vi "TCP IP Connection Tester.vi"() -> ()   [LabVIEW 2024]
panel:
  out "Array":T1(array[cluster])
  in  "port":u16[](array[numeric])
  in  "address":string[](array[string])
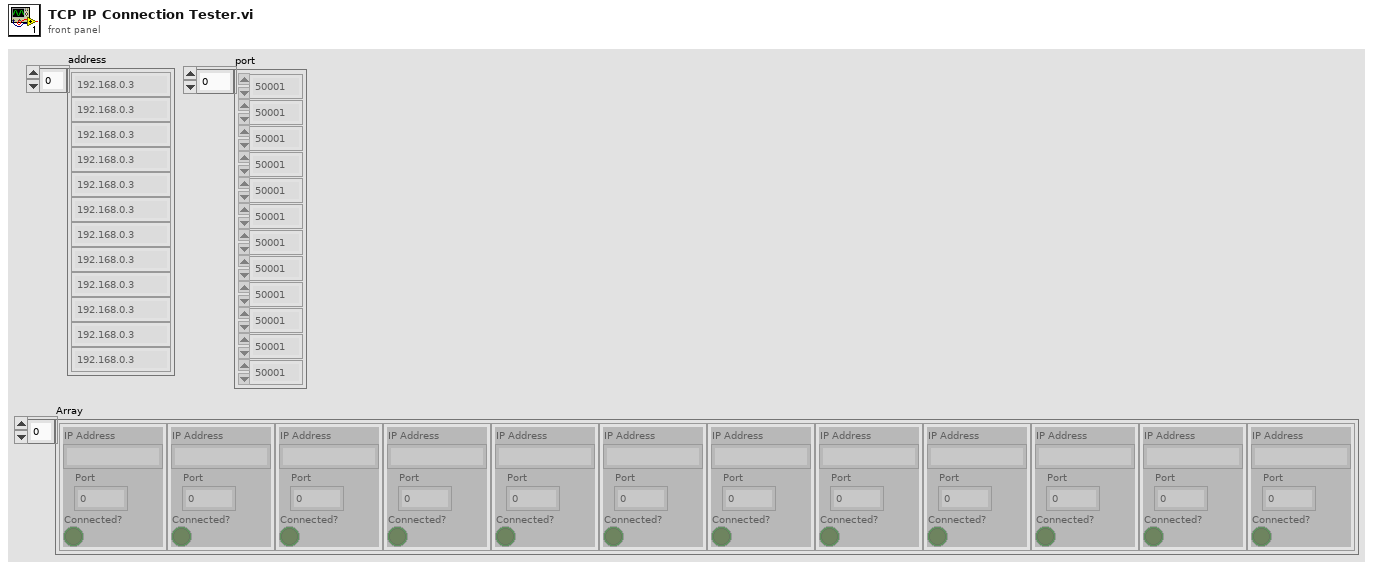
[diagram p1: front panel]
types:
  T1 = cluster{"IP Address":string, "Port":u16, "Connected?":bool}[]
  T2 = cluster{"IP Address":string, "Port":u16, "Connected?":bool}
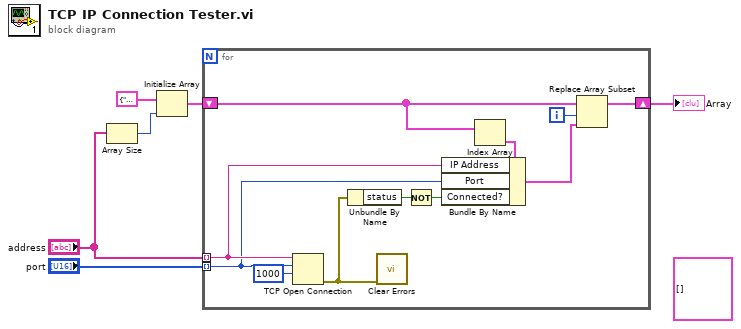
[diagram p0: block diagram]
diagram:
  (unwired) T1 []
  n1 = Array Size(array="address") -> (size(s)=w4:i32)
  n2 = Initialize Array(T2 {"IP Address"="", "Port"=0, "Connected?"=FALSE} ("Cluster"), w4) -> (w2:T1)
  n3 = for {
    tunnel: "port" -> [w14] mode=indexing
    tunnel: "address" -> [w15] mode=indexing
    shift-right: [w10] -> w1
    shift-left: w2 -> [w11]
    i -> [w9]
    n4 = TCP Open Connection(address=w15, remote port or service name=w14, timeout ms (60000)=1000) -> (error out=w7:errorcluster)  [unwired: 2 in, 1 out]
    n5 = Unbundle By Name(w7) -> ("status"=w13:bool)
    n6 = call <vilib>:"Clear Errors.vi"("error in (no error)"=w7) -> ()  [unwired: 5 in, 2 out]
    n7 = Not(x=w13) -> (.not. x?=w12:bool)
    n8 = Index Array(array=w11) -> (element=w16:T2)  [unwired: 1 in]
    n9 = Bundle By Name(cluster=w16, "IP Address"=w15, "Port"=w14, "Connected?"=w12) -> (w8:T2)
    n10 = Replace Array Subset(array=w11, new element=w8, index=w9) -> (w10:T1)
  }
  "Array" <- w1
